vi "Search for packed library.vi"(8 "error in (no error)":errorcluster, 10 "Control Panel Path":path, 11 "Plugin Directory Path":path) -> (0 "error out (no error)":errorcluster, 3 "Control Panel Path Out":path)   [LabVIEW 2020, in "RxnRover.lvlib" / "Plugin Manager.lvlib"]
uses:
  Plugin Manager.lvlib
  <vilib>/Utility/LVLibp/NI_PackedLibraryUtility.lvlib
  logging/logging.lvlib
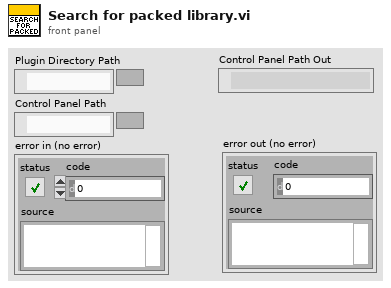
[diagram p1: front panel]
types:
  T1 = enum32{"invalid app kind", "Development System", "Run Time System", "Student Edition", "Embedded LabVIEW", "Evaluation", "Custom"}
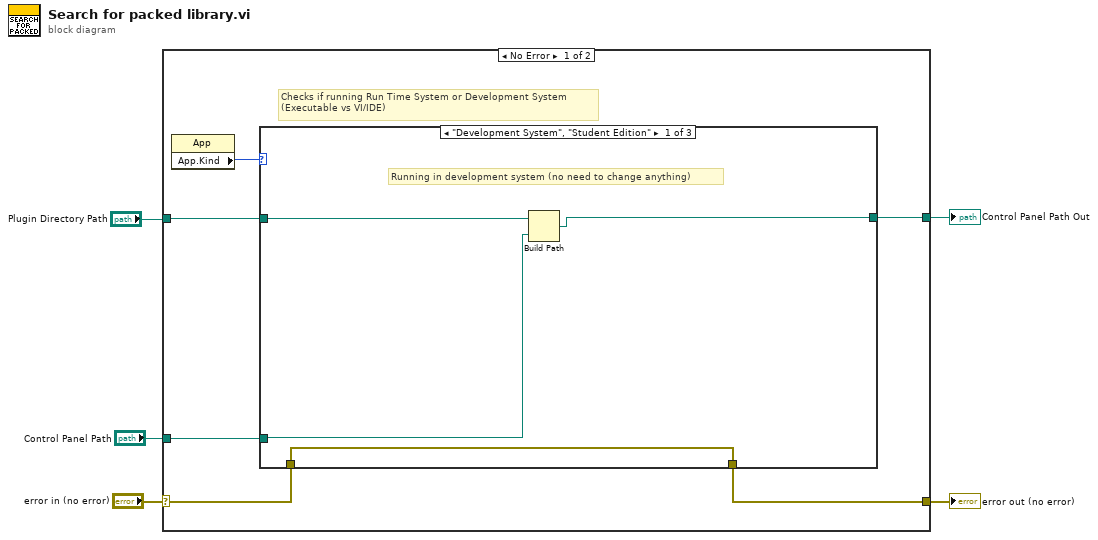
[diagram p0: block diagram]
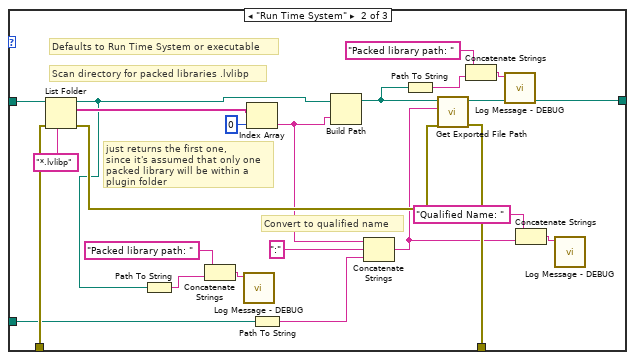
[diagram p2: hidden frame]
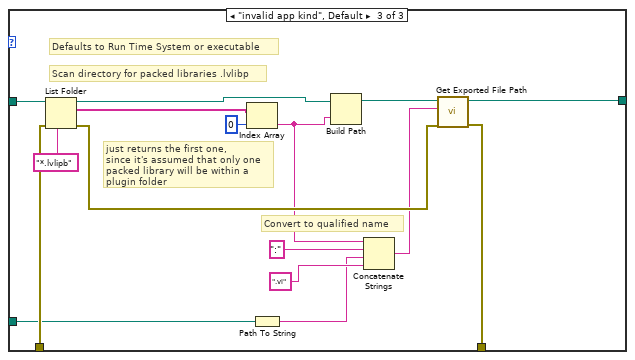
[diagram p3: hidden frame]
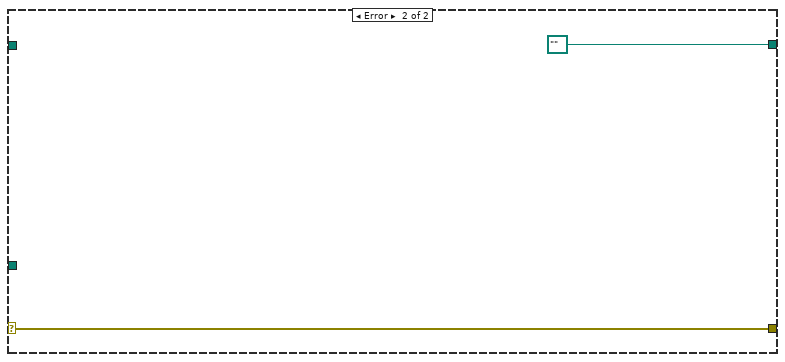
[diagram p4: hidden frame]
diagram:
  n1 = case shown="No Error" "error in (no error)" {
    selector: "error in (no error)" -> [w7 w55]
    tunnel: [w6 w55] -> w4
    tunnel: "Plugin Directory Path" -> [w10 _]
    tunnel: [w9 path "" ("Control Panel Path Out")] -> w2
    tunnel: "Control Panel Path" -> [w8 _]
    frame No Error {
      # "Checks if running Run Time System or Development System\n(Executable vs VI/IDE)"
      n2 = property class="App"() -> ("App.Kind"=w11:T1)  [unwired: 2 in, 2 out]
      n3 = case shown="\"Development System\", \"Student Edition\"" w11 {
        tunnel: w10 -> [w13 w38 w54]
        tunnel: [w12 w32 w48] -> w9
        tunnel: w8 -> [w14 w33 w49]
        tunnel: w7 -> [w15 w37 w53]
        tunnel: [w15 w30 w44] -> w6
        frame "Development System", "Student Edition" {
          # "Running in development system (no need to change anything)"
          n4 = Build Path(base path=w13, name or relative path=w14) -> (appended path=w12:path)
        }
        frame "Run Time System" {
          # "Convert to qualified name"
          # "Defaults to Run Time System or executable"
          # "just returns the first one,\nsince it's assumed that only one\npacked library will be within a plugin folder"
          # "Scan directory for packed libraries .lvlibp"
          n5 = List Folder(path=w38, pattern="*.lvlibp", error in=w37) -> (path out=w17:path, filenames=w35:string[], error out=w31:errorcluster)  [unwired: 1 in, 1 out]
          n6 = Path To String(path=w17) -> (string=w16:string)
          n7 = Concatenate Strings("Packed library path: " ("string"), w16) -> (w19:string)
          n8 = call "Log Message - DEBUG.vi"("Message"=w19) -> ()  [unwired: 10 in, 1 out]
          n9 = Index Array(array=w35, index=0) -> (element=w27:string)
          n10 = Path To String(path=w33) -> (string=w28:string)
          n11 = Build Path(base path=w17, name or relative path=w27) -> (appended path=w21:path)
          n12 = Concatenate Strings(w27, ":" ("string"), w28) -> (w24:string)
          n13 = Path To String(path=w21) -> (string=w20:string)
          n14 = call <vilib>:"Get Exported File Path.vi"("error in (no error)"=w31, "qualified name"=w24, "packed library path"=w21) -> ("error out"=w30:errorcluster, "path"=w32:path)  [unwired: 7 in]
          n15 = Concatenate Strings("Packed library path: " ("string"), w20) -> (w23:string)
          n16 = call "Log Message - DEBUG.vi"("Message"=w23) -> ()  [unwired: 10 in, 1 out]
          n17 = Concatenate Strings("Qualified Name: " ("string"), w24) -> (w26:string)
          n18 = call "Log Message - DEBUG.vi"("Message"=w26) -> ()  [unwired: 10 in, 1 out]
        }
        frame "invalid app kind", Default {
          # "Convert to qualified name"
          # "Defaults to Run Time System or executable"
          # "just returns the first one,\nsince it's assumed that only one\npacked library will be within a plugin folder"
          # "Scan directory for packed libraries .lvlibp"
          n19 = List Folder(path=w54, pattern="*.lvlipb", error in=w53) -> (path out=w47:path, filenames=w51:string[], error out=w45:errorcluster)  [unwired: 1 in, 1 out]
          n20 = Index Array(array=w51, index=0) -> (element=w40:string)
          n21 = Path To String(path=w49) -> (string=w41:string)
          n22 = Build Path(base path=w47, name or relative path=w40) -> (appended path=w46:path)
          n23 = Concatenate Strings(w40, ":" ("string"), w41, ".vi" ("string")) -> (w39:string)
          n24 = call <vilib>:"Get Exported File Path.vi"("error in (no error)"=w45, "qualified name"=w39, "packed library path"=w46) -> ("error out"=w44:errorcluster, "path"=w48:path)  [unwired: 7 in]
        }
      }
    }
    frame Error {
    }
  }
  "Control Panel Path Out" <- w2
  "error out (no error)" <- w4
